vi "Execute Pump OFF.vi"(8 "error in (no error)":errorcluster, 11 "CPC in":refnum<class "3022A.lvclass">) -> (0 "error out":errorcluster, 2 "FP Conc":bool, 3 "CPC out":refnum<class "3022A.lvclass">)   [LabVIEW 2013, in "3022A.lvclass"]
uses:
  3022A/3022A.lvclass
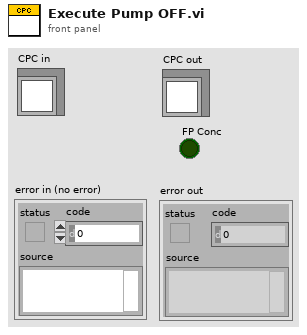
[diagram p1: front panel]
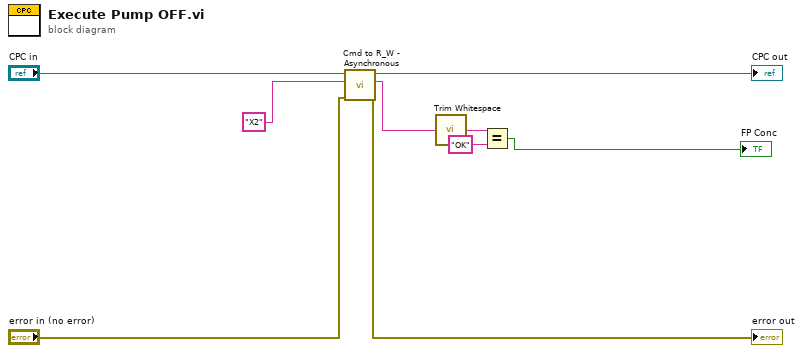
[diagram p0: block diagram]
diagram:
  n1 = call-dynamic "Cmd to R_W - Asynchronous.vi"("error in"="error in (no error)", "write buffer"="X2" ("string"), "Serial IO in"="CPC in") -> ("error out"=→"error out":errorcluster, "read buffer"=w3:string, "Serial IO out"=→"CPC out":refnum<class "3022A.lvclass">)  [unwired: 6 in]
  n2 = call <vilib>:"Trim Whitespace.vi"("string"=w3) -> ("trimmed string"=w2:string)  [unwired: 1 in]
  n3 = Equal?(x=w2, y="OK") -> (x = y?=→"FP Conc":bool)
